vi "Read Record.vi"(8 "error in (no error)":errorcluster, 10 "Account Number":i32, 11 "Simulated Configuration Database Actor in":refnum<class "Configuration Database Actor.lvclass">) -> (0 "error out":errorcluster, 3 "Simulated Configuration Database Actor out":refnum<class "Configuration Database Actor.lvclass">)   [LabVIEW 2019, in "Configuration Database Actor.lvlib" / "Configuration Database Actor.lvclass"]
uses:
  Configuration Database Actor.lvclass
  C:/Program Files (x86)/National Instruments/LabVIEW 2019/vi.lib/ActorFramework/Actor/Actor.lvclass
  <vilib>/ActorFramework/Actor/Actor.lvclass/Actor.ctl
  Configuration Database Actor.lvclass/Configuration Database Actor.ctl
  ATM Controller/ATM Controller Messages/Get DB Record Msg/Get DB Record Msg.lvclass/Get DB Record Msg.ctl
  <vilib>/ActorFramework/Message Enqueuer/Message Enqueuer.lvclass/Message Enqueuer.ctl
  <vilib>/ActorFramework/Message Enqueuer/Enqueue.vi
  ATM Controller/ATM Controller Messages/Get DB Record Msg/Get DB Record Msg.lvclass
  C:/Program Files (x86)/National Instruments/LabVIEW 2019/vi.lib/ActorFramework/Message/Message.lvclass
  <vilib>/ActorFramework/Message Priority Queue/Priority Enqueue.vi
  <vilib>/ActorFramework/Actor/Actor.lvclass
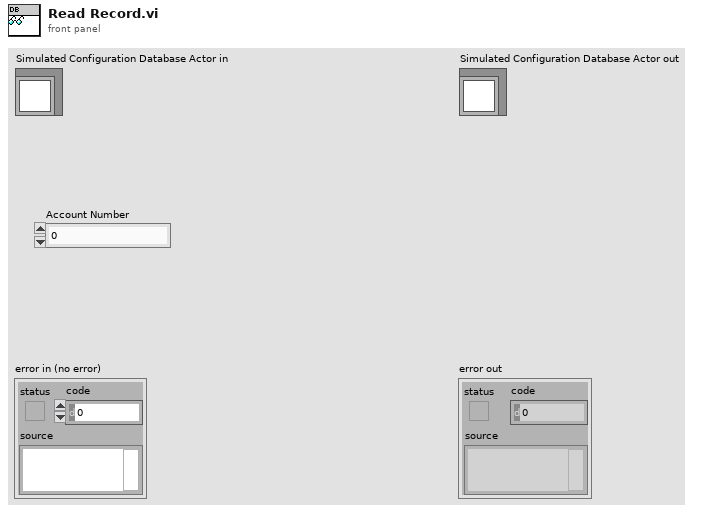
[diagram p1: front panel]
types:
  T1 = typedef "Configuration Database Actor.lvlib/Configuration Database Actor.lvclass/Records -cluster.ctl" = cluster{"Account Number":i32, "First Name":string, "Last Name":string, "Balance":i32}
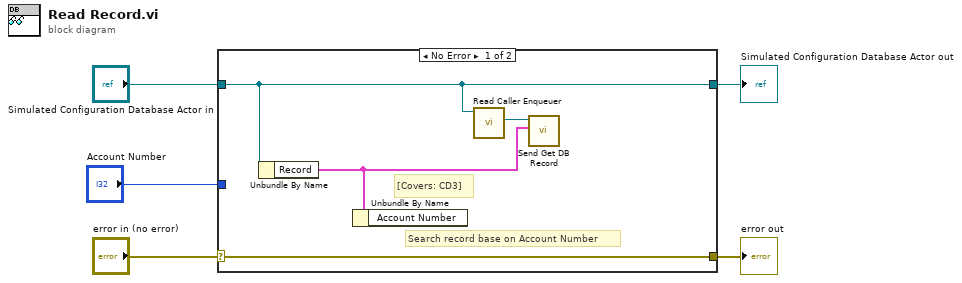
[diagram p0: block diagram]
diagram:
  n1 = case shown="No Error" "error in (no error)" {
    selector: "error in (no error)" -> [w9 w10]
    tunnel: [w9 w10] -> w4
    tunnel: [w8 w11] -> w2
    tunnel: "Simulated Configuration Database Actor in" -> [w8 w11]
    tunnel: "Account Number" -> [_ _]
    frame No Error {
      # "Search record base on Account Number"
      # "[Covers: CD3]"
      n2 = Unbundle By Name(w8) -> ("Record"=w6:T1)
      n3 = Unbundle By Name(w6) -> ()  [unwired: 1 out]
      n4 = call <vilib>:"Read Caller Enqueuer.vi"("Actor"=w8) -> ("Caller Enqueuer"=w7:refnum<class "Message Enqueuer.lvclass">)  [unwired: 10 in]
      n5 = call "Send Get DB Record.vi"("Record"=w6, "Message Enqueuer"=w7) -> ()  [unwired: 8 in, 2 out]
    }
    frame Error {
    }
  }
  "error out" <- w4
  "Simulated Configuration Database Actor out" <- w2
